vi "Set Monitor.vi"(8 "error in":errorcluster, 10 "FP:Monitor":u16, 11 "VI Ref":refnum<vi>) -> (0 "error out":errorcluster, 1 "Disp.Height":i16, 2 "Disp.Width":i16, 3 "Disp.Bounds":T1, 4 "Active Display":u16)   [LabVIEW 2014]
doc: "sets the monitor on which VI front panel will appear, and provides information of that monitor.\nIf the set monitor does not exist, it uses the primary monitor.\n\nWindows: 0 is primary\nOS X: 1 is primary"
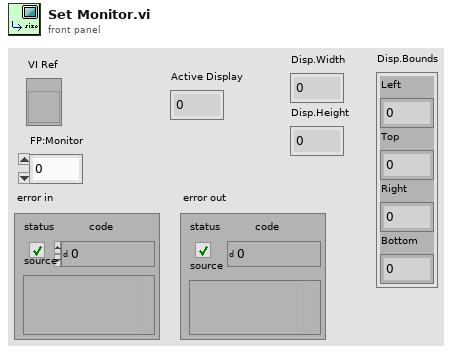
[diagram p1: front panel]
types:
  T1 = cluster{"Left":i16, "Top":i16, "Right":i16, "Bottom":i16}
  T2 = typedef "LVAllMonitorsDisplayTypeDef.ctl" = cluster{"Bounds":cluster{"Left":i16, "Top":i16, "Right":i16, "Bottom":i16}, "Depth":i16}[]
  T3 = cluster{"Bounds":cluster{"Left":i16, "Top":i16, "Right":i16, "Bottom":i16}, "Depth":i16}
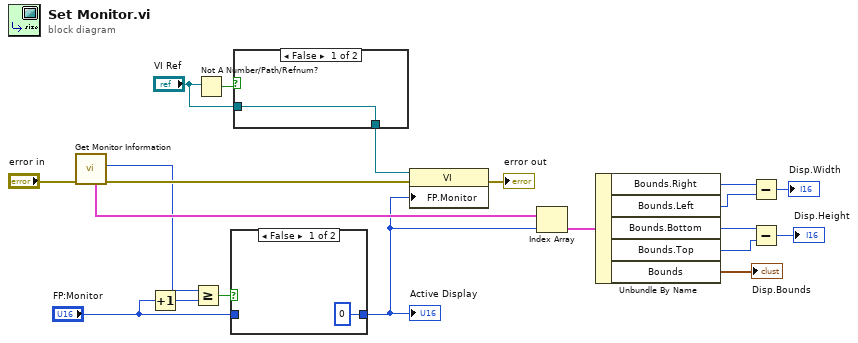
[diagram p0: block diagram]
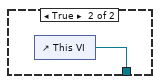
[diagram p3: hidden frame]
diagram:
  n1 = call "Get Monitor Information.vi"("error in"="error in") -> ("error out"=w7:errorcluster, "no. Displays"=w3:i32, "Display:All Monitors"=w9:T2)  [unwired: 6 in, 2 out]
  n2 = Increment(x="FP:Monitor") -> (x+1=w5:u16)
  n3 = Greater Or Equal?(x=w3, y=w5) -> (x >= y?=w6:bool)
  n4 = Not A Number/Path/Refnum?(number/path/refnum="VI Ref") -> (NaN/Path/Refnum?=w17:bool)
  n5 = case shown="False" w6 {
    tunnel: "FP:Monitor" -> [_ w22]
    tunnel: [u16 0 ("FP:Monitor") w22] -> w1
    frame False {
    }
    frame True {
    }
  }
  "Active Display" <- w1
  n6 = case shown="False" w17 {
    tunnel: "VI Ref" -> [w23 _]
    tunnel: [w23 w24] -> w16
    frame False {
    }
    frame True {
      n7 = control-ref of="This VI"() -> (w24:refnum<vi>)
    }
  }
  n8 = property class="VI"(reference=w16, error in=w7, "FP.Monitor"=w1) -> (error out=→"error out":errorcluster)  [unwired: 1 out]
  n9 = Index Array(array=w9, index=w1) -> (element=w20:T3)
  n10 = Unbundle By Name(w20) -> ("Bounds.Right"=w15:i16, "Bounds.Left"=w14:i16, "Bounds.Bottom"=w12:i16, "Bounds.Top"=w11:i16, "Bounds"=→"Disp.Bounds":T1)
  n11 = Subtract(x=w15, y=w14) -> (x-y=→"Disp.Width":i16)
  n12 = Subtract(x=w12, y=w11) -> (x-y=→"Disp.Height":i16)
